vi "SmootherPath.vi"(4 "ignoreBall?":bool, 6 "ball":T1, 8 "Robot in":T2={"id"=0, "function"=enum."Attacker", "x"=0.0, "y"=0.0, "orientation"=0.0, "v_tangent"=0.0, "v_normal"=0.0, "v_ang"=0.0, "kick_x"=0.0, "kick_z"=0.0, "dribble"=FALSE, "Timestamp"=timestamp(0 s since 1904-01-01), "estimatives"={"est_v_tangent"=0.0, "est_v_normal"=0.0, "est_vx"=0.0, "est_vy"=0.0, "Pos Robot Est"=[]}, "dest_x_kick"=0.0, "dest_y_kick"=0.0, "Gap Coord"=[], "States"=enum."GoToTangent", "Path "=[], "Path  Smooth"=[], "Dest"=[], "vx_desired"=0.0, "vy_desired"=0.0, "slowBehavior"=FALSE, "VSSStates"=enum."Pass"}, 9 "SmoothPath":dbl[][](array[numeric]), 10 "enemy_robots":T2[](array[typedef]), 11 "our_robots":T2[](array[typedef])) -> (1 "SmootherPath":dbl[][](array[numeric]))   [LabVIEW 2023]
uses:
  Vision_class/Old vision/Controls/AI Robot.ctl
  Vision_class/Old vision/Controls/Functions Enum.ctl
  Vision_class/Old vision/Controls/AttackerStates.ctl
  Vision_class/Old vision/Controls/PathDests.ctl
  Vision_class/Old vision/Controls/PathDest.ctl
  Navigation/VSSNavigation/VSSAttackerStates.ctl
  Vision_class/Old vision/SSL Detection Frame Simple Estimator Cameras VelCmd Folder/Core/AI Ball.ctl
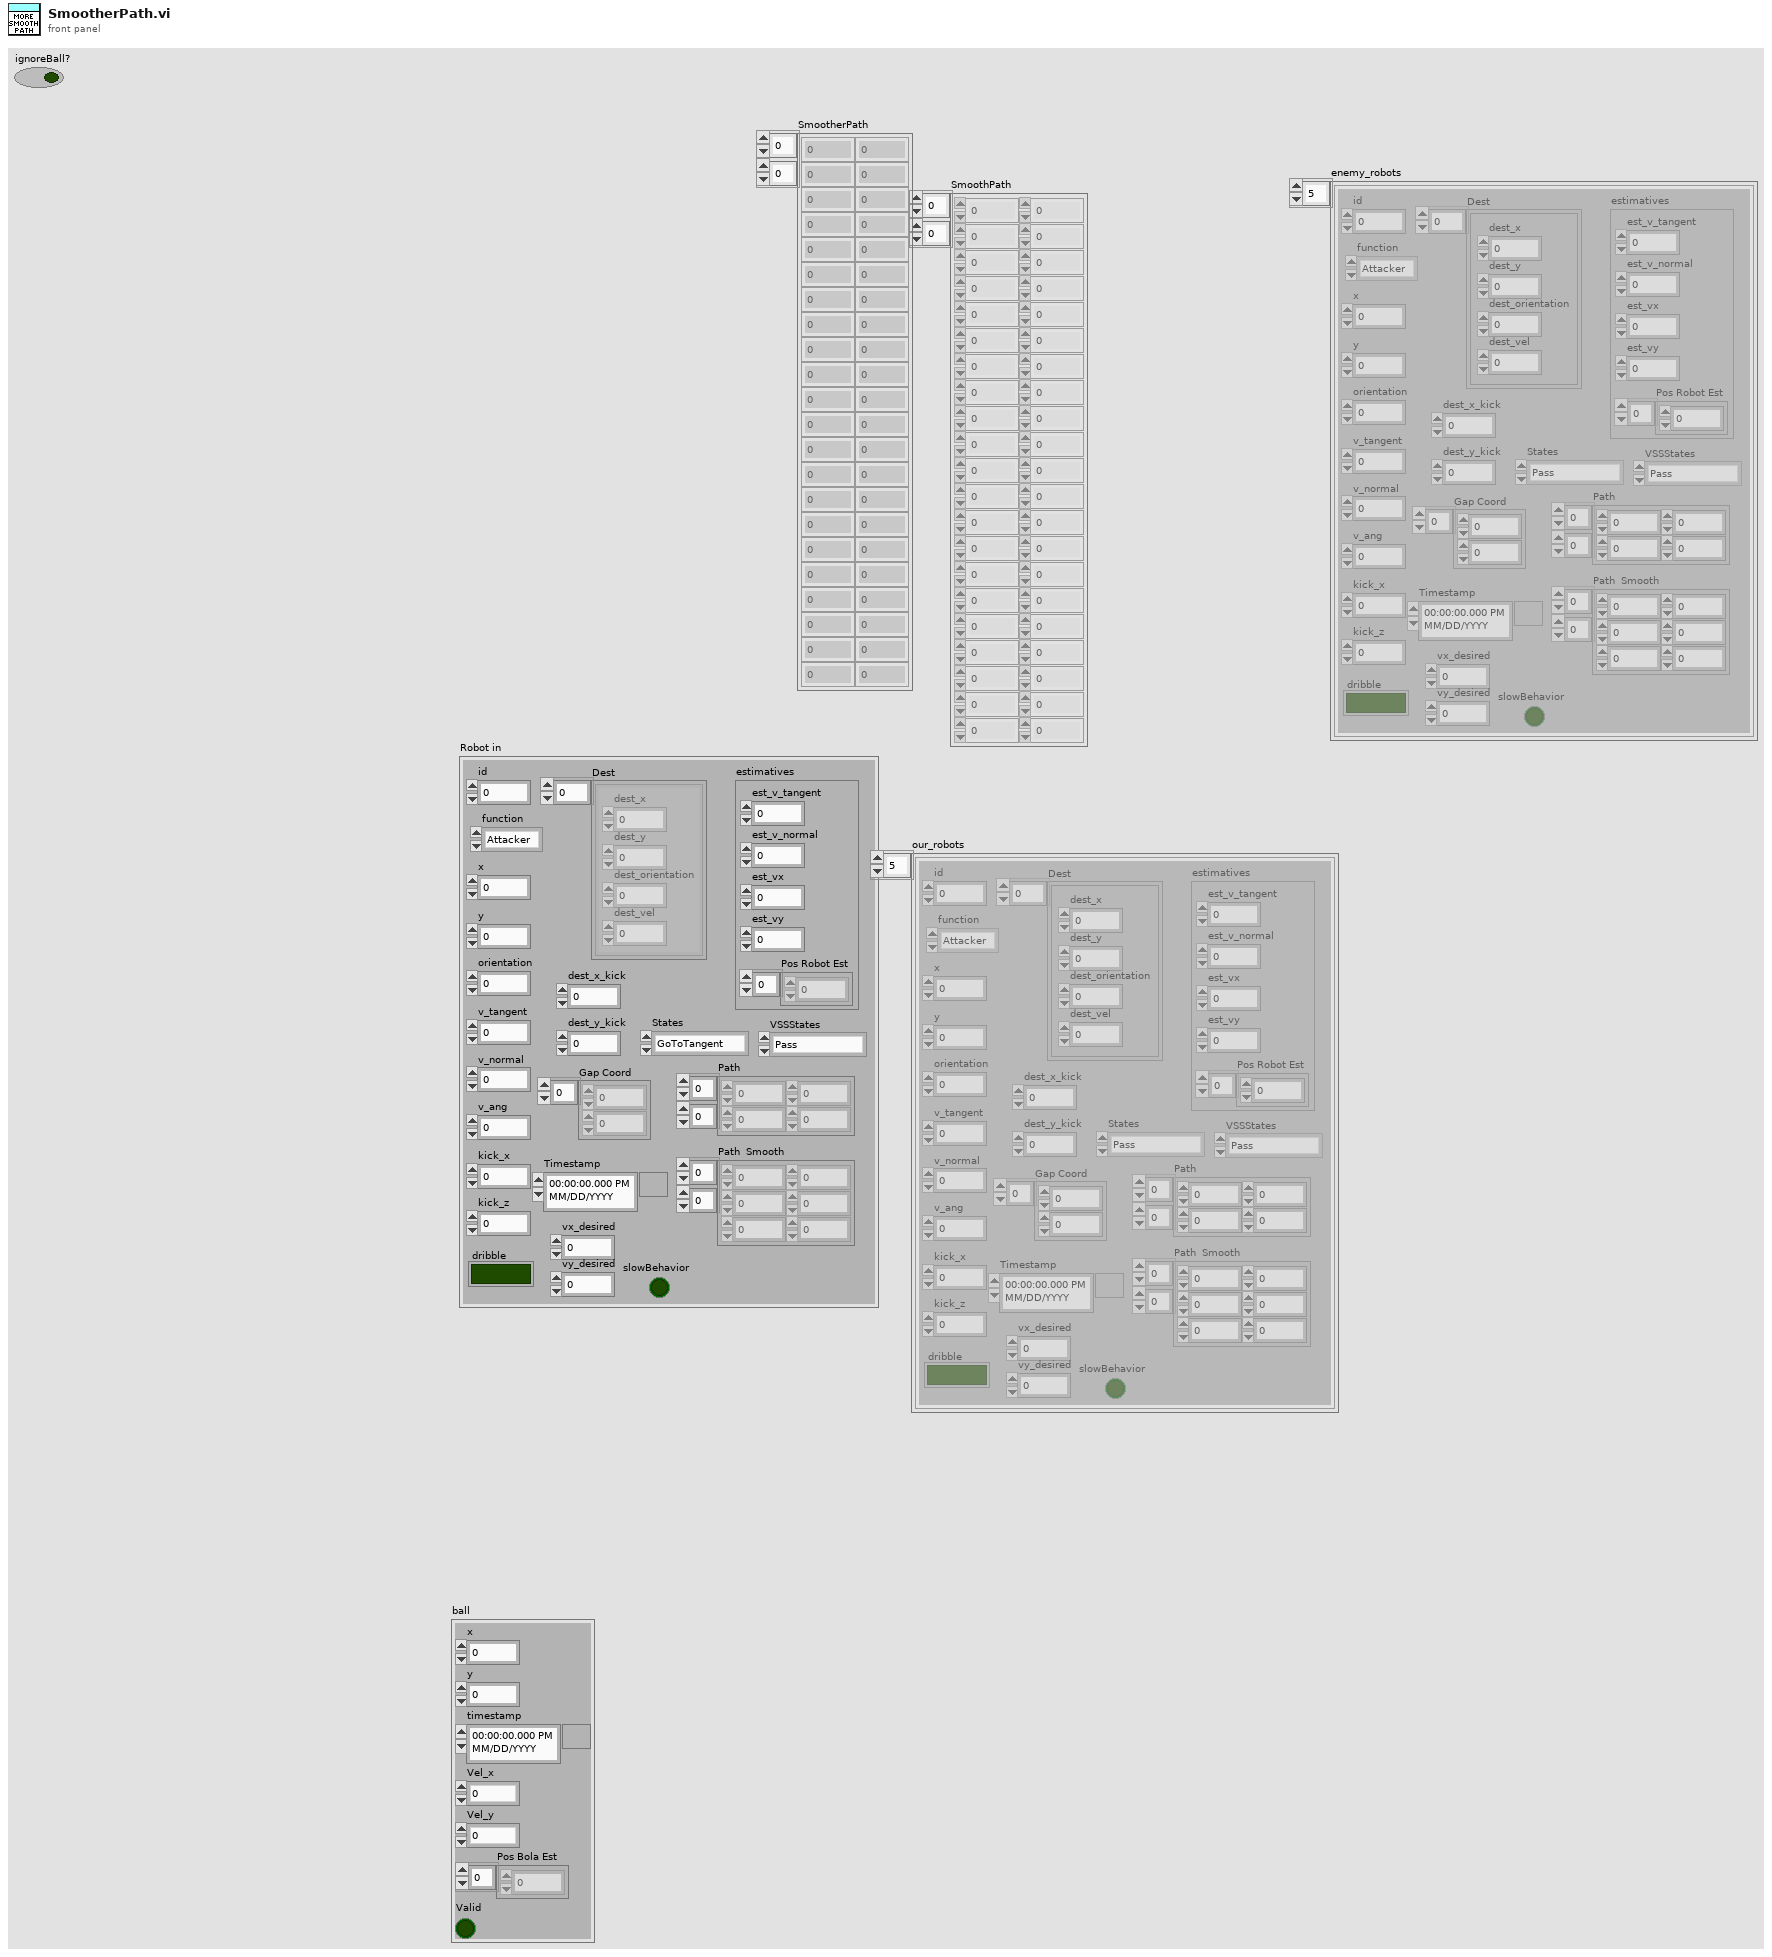
[diagram p1: front panel]
types:
  T1 = typedef "AI Ball.ctl" = cluster{"x":dbl, "y":dbl, "timestamp":timestamp, "Vel_x":dbl, "Vel_y":dbl, "Pos Bola Est":dbl[], "Valid":bool}
  T2 = typedef "AI Robot.ctl" = cluster{"id":u32, "function":T3, "x":dbl, "y":dbl, "orientation":dbl, "v_tangent":dbl, "v_normal":dbl, "v_ang":dbl, "kick_x":dbl, "kick_z":dbl, "dribble":bool, "Timestamp":timestamp, "estimatives":cluster{"est_v_tangent":dbl, "est_v_normal":dbl, "est_vx":dbl, "est_vy":dbl, "Pos Robot Est":dbl[]}, "dest_x_kick":dbl, "dest_y_kick":dbl, "Gap Coord":dbl[], "States":T4, "Path ":dbl[][], "Path  Smooth":dbl[][], "Dest":T5, "vx_desired":dbl, "vy_desired":dbl, "slowBehavior":bool, "VSSStates":T7}
  T3 = typedef "Functions Enum.ctl" = enum16{"2nd Striker", "Attacker", "Goalie", "Defender", "Striker", "Goto 0", "Dummy", "Kicker", "ZigZag 0", "ZigZag 1", "ZigZag 2", "ZigZag 3", "ZigZag 4", "ZigZag 5", "ZigZag 6", "ZigZag 7", "ZigZag 8", ""}
  T4 = typedef "AttackerStates.ctl" = enum16{"Pass", "GoToTangent", "BallGetting", "GoToKick", ""}
  T5 = typedef "PathDests.ctl" = T6[]
  T6 = typedef "PathDest.ctl" = cluster{"dest_x":dbl, "dest_y":dbl, "dest_orientation":dbl, "dest_vel":dbl}
  T7 = typedef "VSSAttackerStates.ctl" = enum16{"Pass", "GoToTangent", "BallGetting", "GoToKick", "Rotate anti-clockwise", "Rotate Clockwise", ""}
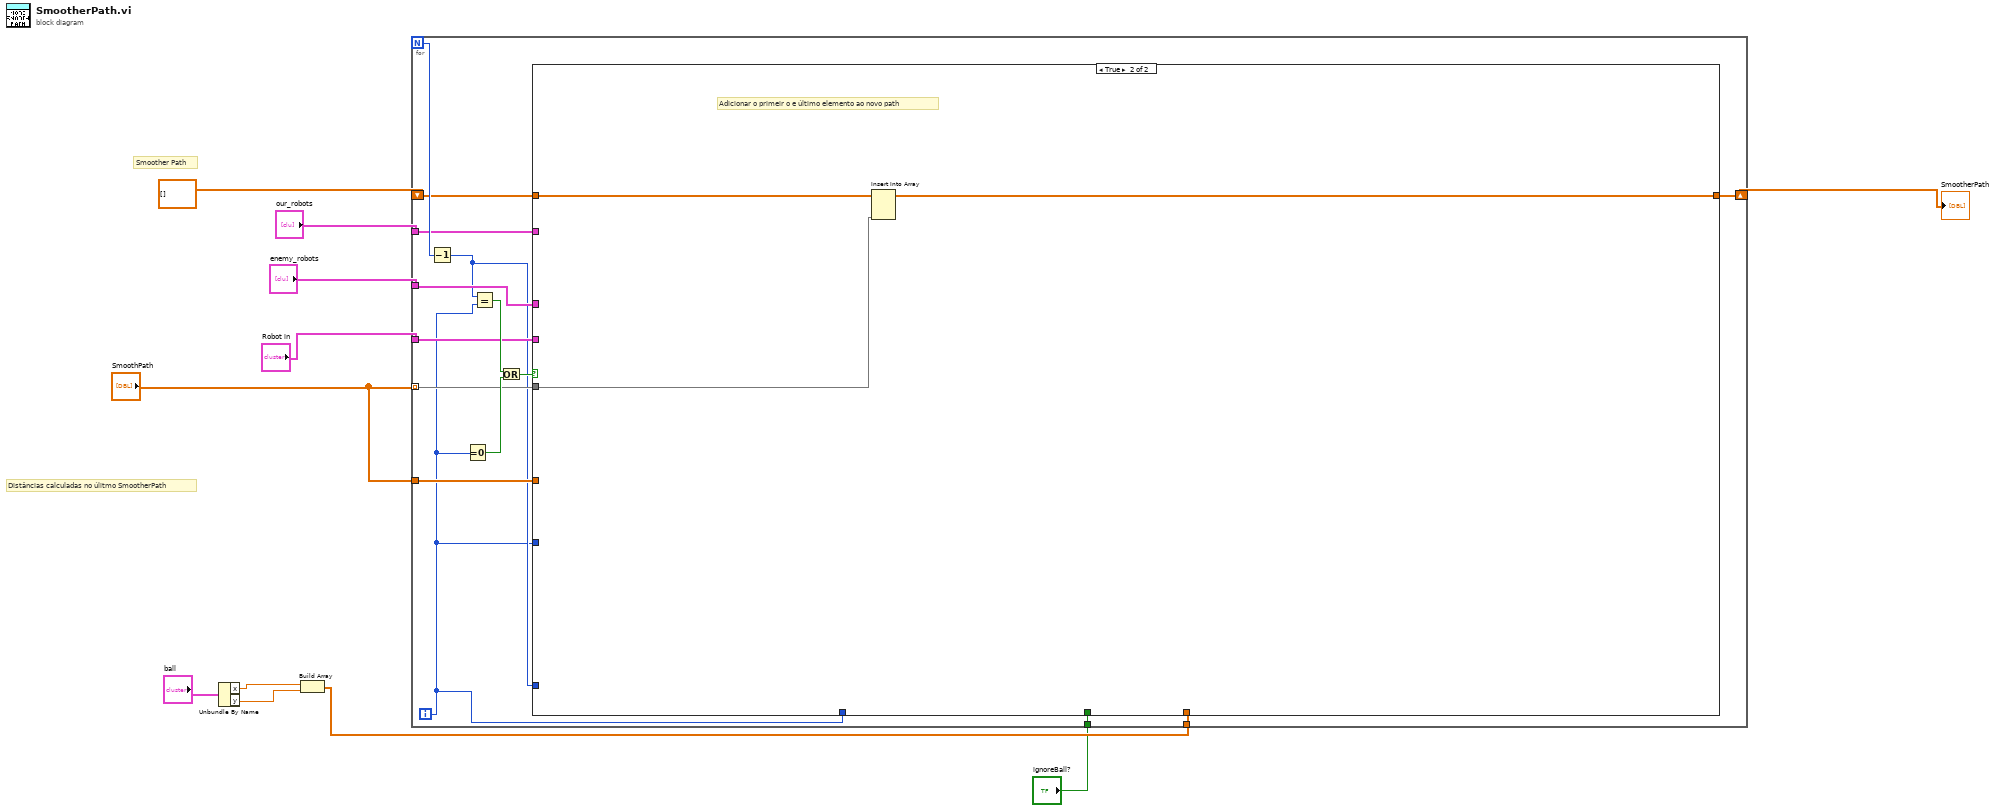
[diagram p0: block diagram]
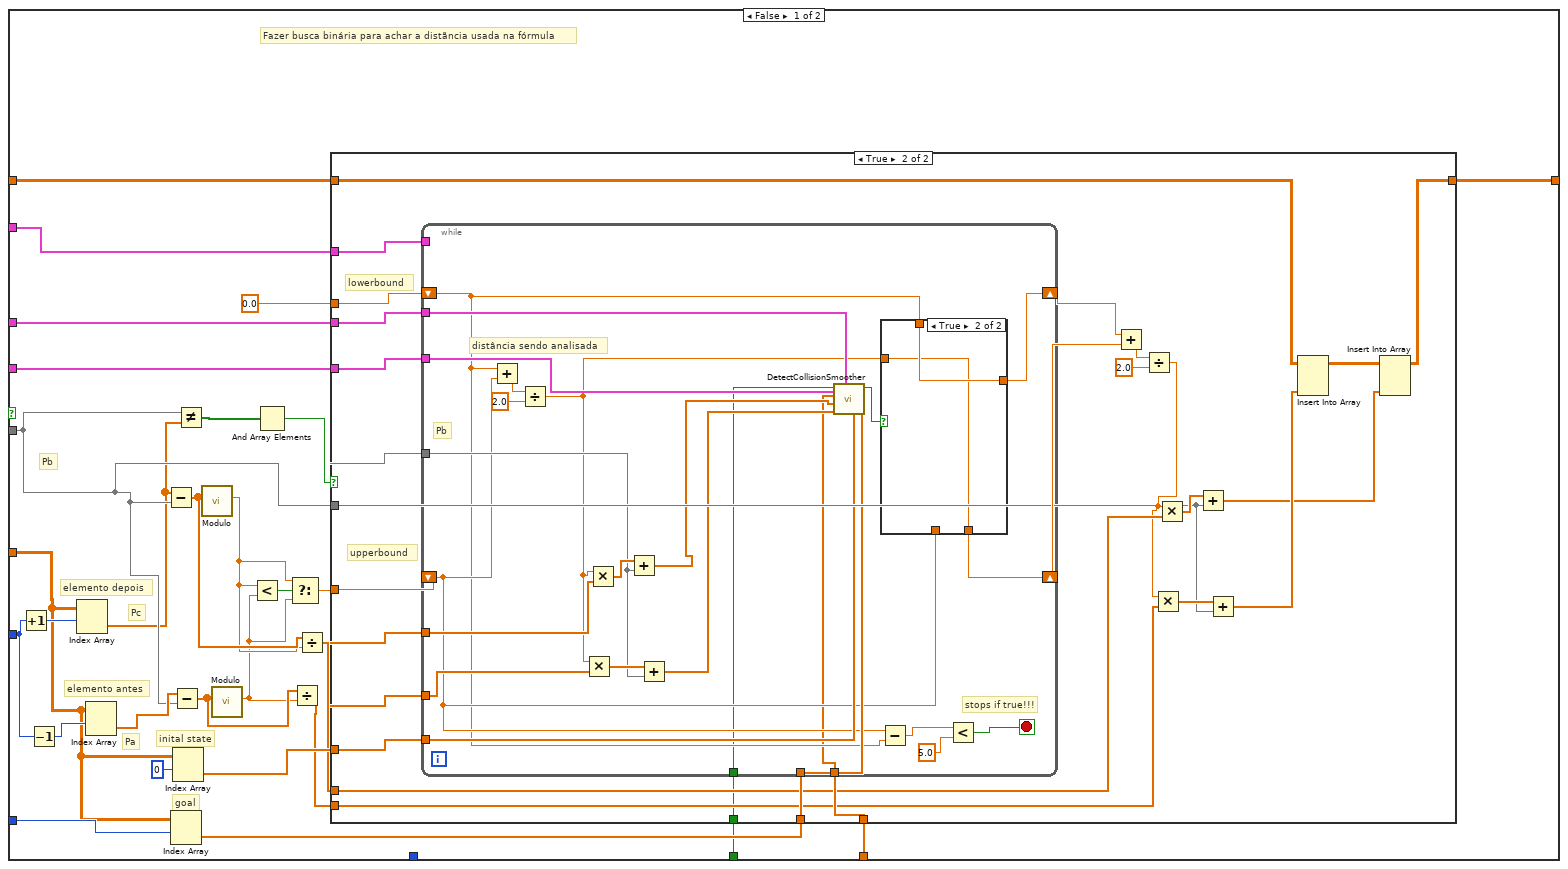
[diagram p2: hidden frame]
diagram:
  # "Distâncias calculadas no úlitmo SmootherPath"
  # "Smoother Path"
  n1 = Unbundle By Name("ball") -> ("x"=w10:dbl, "y"=w9:dbl)
  n2 = Build Array(w10, w9) -> (w4:dbl[])
  n3 = for {
    N -> [w26]
    tunnel: "SmoothPath" -> [w21] mode=indexing
    shift-right: [w20] -> w2
    shift-left: dbl[][] [] ("Path") -> [w23]
    tunnel: "SmoothPath" -> [w19]
    tunnel: "our_robots" -> [w18]
    tunnel: "enemy_robots" -> [w17]
    tunnel: "Robot in" -> [w16]
    tunnel: w4 -> [w14]
    tunnel: "ignoreBall?" -> [w12]
    i -> [w13]
    n4 = Decrement(x=w26) -> (x-1=w15:i32)
    n5 = Equal To 0?(x=w13) -> (x = 0?=w24:bool)
    n6 = Equal?(x=w15, y=w13) -> (x = y?=w25:bool)
    n7 = Or(x=w25, y=w24) -> (x .or. y?=w22:bool)
    n8 = case shown="True" w22 {
      tunnel: w23 -> [w37 w111]
      tunnel: w21 -> [w31 w110]
      tunnel: [w36 w109] -> w20
      tunnel: w19 -> [w32 _]
      tunnel: w13 -> [w34 _]
      tunnel: w18 -> [w46 _]
      tunnel: w17 -> [w45 _]
      tunnel: w16 -> [w44 _]
      tunnel: w15 -> [w42 _]
      tunnel: w14 -> [w39 _]
      tunnel: w13 -> [_ _]
      tunnel: w12 -> [w27 _]
      frame False {
        # "Pa"
        # "Pc"
        # "Pb"
        # "goal"
        # "inital state"
        # "elemento antes"
        # "elemento depois"
        # "Fazer busca binária para achar a distãncia usada na fórmula"
        n9 = Increment(x=w34) -> (x+1=w55:i32)
        n10 = Decrement(x=w34) -> (x-1=w54:i32)
        n11 = Index Array(array=w32, index (row)=w55) -> (element=w30:dbl[])  [unwired: 1 in]
        n12 = Index Array(array=w32, index (row)=w54) -> (element=w33:dbl[])  [unwired: 1 in]
        n13 = Subtract(x=w30, y=w31) -> (x-y=w50:dbl[])
        n14 = Index Array(array=w32, index (row)=w42) -> (element=w40:dbl[])  [unwired: 1 in]
        n15 = Subtract(x=w33, y=w31) -> (x-y=w48:dbl[])
        n16 = Index Array(array=w32, index (row)=0) -> (element=w41:dbl[])  [unwired: 1 in]
        n17 = Not Equal?(x=w31, y=w30) -> (x != y?=w29:bool[])
        n18 = call "Modulo.vi"("2D vector"=w50) -> ("Modulo"=w49:dbl)  [unwired: 10 in]
        n19 = call "Modulo.vi"("2D vector"=w48) -> ("Modulo"=w47:dbl)  [unwired: 10 in]
        n20 = Less?(x=w49, y=w47) -> (x < y?=w52:bool)
        n21 = And Array Elements(Boolean array=w29) -> (logical AND=w28:bool)
        n22 = Select(t=w49, s=w52, f=w47) -> (s? t:f=w51:dbl)
        n23 = Divide(x=w48, y=w47) -> (x/y=w35:dbl[])
        n24 = Divide(x=w50, y=w49) -> (x/y=w38:dbl[])
        n25 = case shown="True" w28 {
          tunnel: 0.0 -> [_ w80]
          tunnel: w51 -> [_ w79]
          tunnel: w46 -> [_ w78]
          tunnel: w45 -> [_ w77]
          tunnel: w44 -> [_ w76]
          tunnel: w41 -> [_ w75]
          tunnel: w40 -> [_ w74]
          tunnel: w39 -> [_ w73]
          tunnel: w38 -> [_ w66]
          tunnel: w37 -> [w56 w65]
          tunnel: [w56 w63] -> w36
          tunnel: w35 -> [_ w62]
          tunnel: w31 -> [_ w60]
          tunnel: w27 -> [_ w57]
          frame False {
          }
          frame True {
            # "upperbound"
            # "lowerbound"
            n26 = while {
              shift-right: [w87] -> w70
              shift-left: w80 -> [w85]
              shift-right: [w86] -> w69
              shift-left: w79 -> [w88]
              tunnel: w60 -> [w95]
              tunnel: w62 -> [w99]
              tunnel: w66 -> [w98]
              tunnel: w78 -> [_]
              tunnel: w77 -> [w94]
              tunnel: w76 -> [w93]
              tunnel: w75 -> [w92]
              tunnel: w74 -> [w91]
              tunnel: w73 -> [w82]
              tunnel: w57 -> [w81]
              stop <- w102 stop-if-true
              # "distância sendo analisada"
              # "Pb"
              # "stops if true!!!"
              n27 = Add(x=w85, y=w88) -> (x+y=w101:dbl)
              n28 = Divide(x=w101, y=2.0) -> (x/y=w89:dbl)
              n29 = Multiply(x=w89, y=w99) -> (x*y=w97:dbl[])
              n30 = Multiply(x=w89, y=w98) -> (x*y=w96:dbl[])
              n31 = Add(x=w96, y=w95) -> (x+y=w84:dbl[])
              n32 = Add(x=w97, y=w95) -> (x+y=w83:dbl[])
              n33 = call "DetectCollisionSmoother.vi"("Goal"=w91, "Initial State"=w92, "enemy_robots"=w94, "Robot in"=w93, "SegmentPointB"=w83, "SegmentPointA"=w84, "ball"=w82, "ignoreBall?"=w81) -> ("Is there colision?"=w90:bool)  [unwired: 3 in]
              n34 = Subtract(x=w88, y=w85) -> (x-y=w104:dbl)
              n35 = case shown="True" w90 {
                tunnel: w89 -> [w106 w107]
                tunnel: w85 -> [_ w108]
                tunnel: w88 -> [w105 _]
                tunnel: [w106 w108] -> w87
                tunnel: [w105 w107] -> w86
                frame False {
                }
                frame True {
                }
              }
              n36 = Less?(x=w104, y=5.0) -> (x < y?=w102:bool)
            }
            n37 = Add(x=w70, y=w69) -> (x+y=w72:dbl)
            n38 = Divide(x=w72, y=2.0) -> (x/y=w61:dbl)
            n39 = Multiply(x=w61, y=w62) -> (x*y=w68:dbl[])
            n40 = Multiply(x=w61, y=w66) -> (x*y=w67:dbl[])
            n41 = Add(x=w67, y=w60) -> (x+y=w58:dbl[])
            n42 = Add(x=w68, y=w60) -> (x+y=w59:dbl[])
            n43 = Insert Into Array(array=w65, new element=w59) -> (w64:dbl[][])  [unwired: 2 in]
            n44 = Insert Into Array(array=w64, new element=w58) -> (w63:dbl[][])  [unwired: 2 in]
          }
        }
      }
      frame True {
        # "Adicionar o primeir o e último elemento ao novo path"
        n45 = Insert Into Array(array=w111, new element=w110) -> (w109:dbl[][])  [unwired: 2 in]
      }
    }
  }
  "SmootherPath" <- w2
